vi "Register to Container Events.vi"(8 "error in (no error)":errorcluster, 11 "GUI Container in":refnum<class "GUI Container.lvclass">) -> (0 "error out":errorcluster, 2 "Event Registration Refnum":refnum<event-registration>, 3 "GUI Container out":refnum<class "GUI Container.lvclass">)   [LabVIEW 2023, in "GUI Views.lvlib" / "GUI Container.lvclass"]
doc: "This method must be used in the \"Actor Core.vi\" of the subclass of the \"GUI Container Actor\". It will register two events created by the \"GUI Container Actor\", one can be used to exit the helper loop if present, and the other can be used to allow the optional event loop to receive the views contained by the \"GUI Container Actor\". Calling this method is optional. See the examples for an illustration of its usage."
uses:
  GUI Container.lvclass
  GUI Container.lvclass/GUI Container.ctl
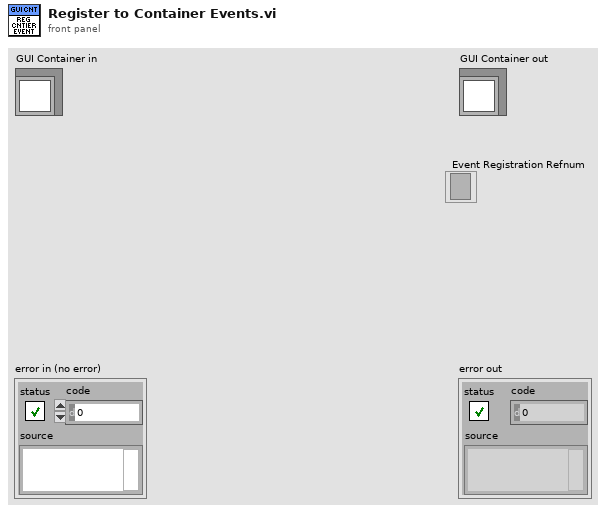
[diagram p1: front panel]
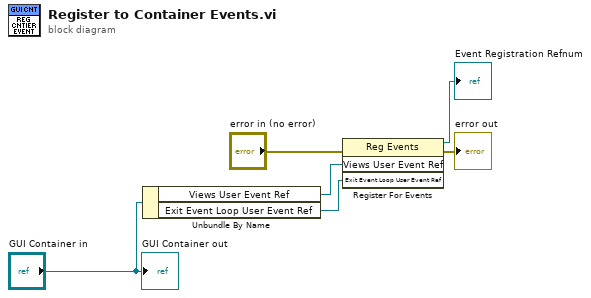
[diagram p0: block diagram]
diagram:
  n1 = Unbundle By Name("GUI Container in") -> ("Views User Event Ref"=w3:refnum<user-event>, "Exit Event Loop User Event Ref"=w2:refnum<user-event>)
  n2 = register-events(error in="error in (no error)", w3, w2) -> (reference out=→"Event Registration Refnum":refnum<event-registration>, error out=→"error out":errorcluster)  [unwired: 1 in]
  "GUI Container out" <- "GUI Container in"
